vi "FileFolderPathToJson.vi"(8 "error in (no error)":errorcluster, 9 "Paths in":T1[](array[typedef]), 10 "Path":path, 11 "head in":refnum<data-value>) -> (0 "error out":errorcluster, 1 "Paths out":T1[](array[typedef]), 2 "String":string, 3 "head out":refnum<data-value>)   [LabVIEW 2017]
uses:
  JsonConverters/Helpers/DirectoryMetadata/DirectoryMetadata.lvclass
  JsonConverters/SourceJsonPaths.ctl
  PathConfiguration.vi
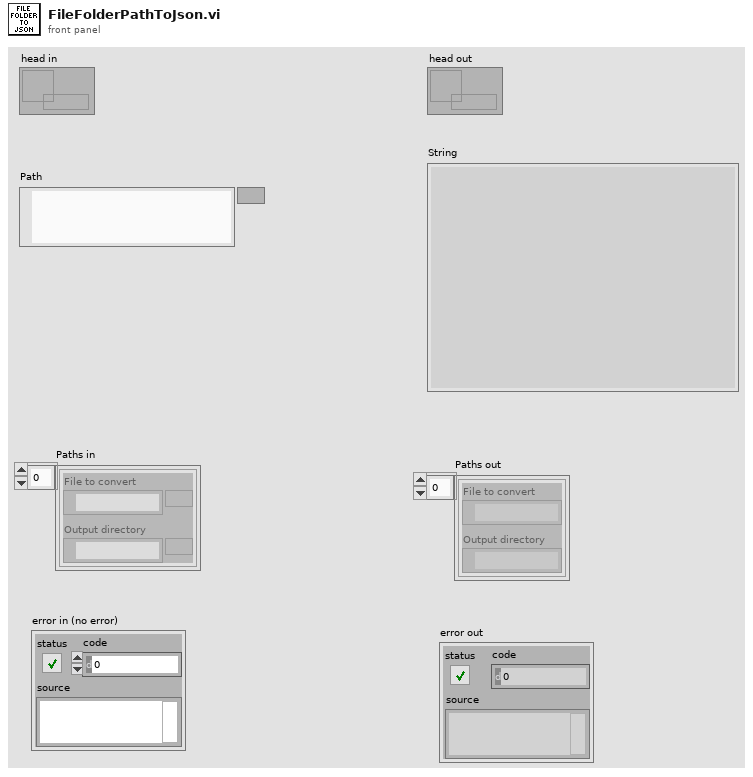
[diagram p1: front panel]
types:
  T1 = typedef "SourceJsonPaths.ctl" = cluster{"File to convert":path, "Output directory":path}
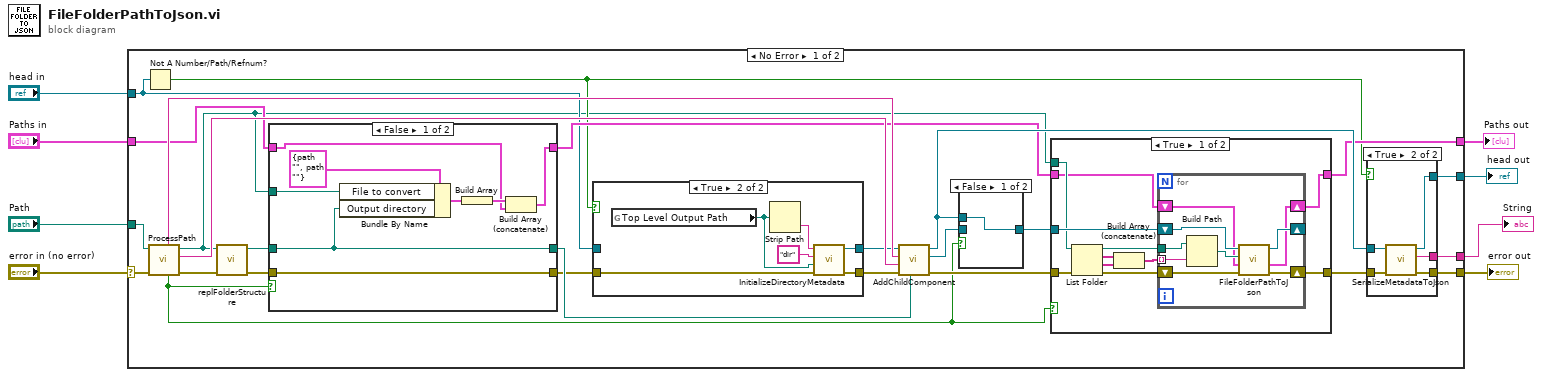
[diagram p0: block diagram]
diagram:
  n1 = case shown="No Error" "error in (no error)" {
    selector: "error in (no error)" -> [w29 w87]
    tunnel: "Path" -> [w34 _]
    tunnel: "head in" -> [w13 w86]
    tunnel: [w26 w87] -> w7
    tunnel: [w28 w86] -> w6
    tunnel: [w25 _] -> w5
    tunnel: "Paths in" -> [w21 w85]
    tunnel: [w23 w85] -> w1
    frame No Error {
      n2 = Not A Number/Path/Refnum?(number/path/refnum=w13) -> (NaN/Path/Refnum?=w14:bool)
      n3 = call "ProcessPath.vi"("error in (no error)"=w29, "path in"=w34) -> ("error out"=w22:errorcluster, "Type"=w33:string, "path out"=w9:path, "Is Directory?"=w17:bool, "File/Folder name"=w32:string)  [unwired: 5 in]
      n4 = call "replFolderStructure.vi"("error in (no error)"=w22, "File to convert"=w9) -> ("error out"=w18:errorcluster, "rep path"=w19:path)  [unwired: 8 in]
      n5 = case shown="False" w17 {
        tunnel: w9 -> [w56 _]
        tunnel: w18 -> [w53 w62]
        tunnel: [w53 w62] -> w11
        tunnel: w21 -> [w55 w61]
        tunnel: [w54 w61] -> w20
        tunnel: w19 -> [w52 w60]
        tunnel: [w52 w60] -> w16
        frame False {
          n6 = Bundle By Name(cluster=T1 {"File to convert"=path "", "Output directory"=path ""} ("TimeStamp"), "File to convert"=w56, "Output directory"=w52) -> (w59:T1)
          n7 = Build Array(w59) -> (w58:T1[])
          n8 = Build Array (concatenate)(w58, w55) -> (w54:T1[])
        }
        frame True {
        }
      }
      n9 = case shown="True" w14 {
        tunnel: w13 -> [w36 _]
        tunnel: [w36 w40] -> w12
        tunnel: w11 -> [w35 w39]
        tunnel: [w35 w38] -> w10
        frame False {
        }
        frame True {
          n10 = global read "PathConfiguration.vi" "Top Level Output Path"() -> (w37:path)
          n11 = Strip Path(path=w37) -> (name=w41:string)  [unwired: 1 out]
          n12 = call "InitializeDirectoryMetadata.vi"("Error in"=w39, "Path"=w37, "Type"="dir", "ID"=w41) -> ("Error out"=w38:errorcluster, "DirectoryMetadata instance"=w40:refnum<data-value>)  [unwired: 6 in]
        }
      }
      n13 = call "AddChildComponent.vi"("Path"=w16, "error in (no error)"=w10, "Type"=w33, "ID"=w32, "head in"=w12) -> ("error out"=w30:errorcluster, "child ref"=w15:refnum<data-value>, "head out"=w24:refnum<data-value>)  [unwired: 4 in]
      n14 = case shown="False" w17 {
        tunnel: [w43 w44] -> w31
        tunnel: w15 -> [_ w44]
        tunnel: w24 -> [w43 _]
        frame False {
        }
        frame True {
        }
      }
      n15 = case shown="True" w17 {
        tunnel: w30 -> [w73 w84]
        tunnel: w9 -> [w69 _]
        tunnel: [w71 w84] -> w27
        tunnel: w31 -> [w70 _]
        tunnel: w20 -> [w66 w83]
        tunnel: [w67 w83] -> w23
        frame True {
          n16 = List Folder(path=w69, error in=w73) -> (path out=w68:path, filenames=w65:string[], folder names=w64:string[], error out=w72:errorcluster)  [unwired: 2 in]
          n17 = Build Array (concatenate)(w65, w64) -> (w63:string[])
          n18 = for {
            shift-right: [w76] -> w71
            shift-left: w72 -> [w77]
            tunnel: w63 -> [w81] mode=indexing
            tunnel: w68 -> [w82]
            shift-right: [w79] -> _
            shift-left: w70 -> [w80]
            shift-right: [w74] -> w67
            shift-left: w66 -> [w75]
            n19 = Build Path(base path=w82, name or relative path=w81) -> (appended path=w78:path)
            n20 = call "FileFolderPathToJson.vi"("error in (no error)"=w77, "Paths in"=w75, "Path"=w78, "head in"=w80) -> ("error out"=w76:errorcluster, "Paths out"=w74:T1[], "head out"=w79:refnum<data-value>)  [unwired: 4 in, 1 out]
          }
        }
        frame False {
        }
      }
      n21 = case shown="True" w14 {
        tunnel: [w46 w51] -> w28
        tunnel: w27 -> [w45 w50]
        tunnel: [w45 w49] -> w26
        tunnel: [_ w48] -> w25
        tunnel: w24 -> [w46 w47]
        frame False {
        }
        frame True {
          n22 = call "SerializeMetadataToJson.vi"("error in (no error)"=w50, "head in"=w47) -> ("error out"=w49:errorcluster, "Serialized String"=w48:string, "head out"=w51:refnum<data-value>)  [unwired: 7 in]
        }
      }
    }
    frame Error {
    }
  }
  "error out" <- w7
  "head out" <- w6
  "String" <- w5
  "Paths out" <- w1
